vi "PPWV Partial Pressure of Water Vapor (Pa) Pressure Dependent.vi"(1 "Pressure":dbl[unit], 2 "Tceg":dbl[unit], 3 "RH":dbl) -> (0 "PPWV":dbl[unit])   [LabVIEW 2018]
panel:
  out "RH":dbl(knob) scale=0.0..10.0
  out "Pressure":dbl[unit](knob)
  out "PPWV\nPartial Presure of Water Vapor (Pa) Pressure Dependent;\nPPWV=(SVP*RH)/100;":dbl[unit](knob)
  out "Temprature Of Input Air\nKelvin Degree":dbl[unit](slide) scale=273.0..373.0
  out "Tk":dbl[unit]
  out "Temprature Of Input Air\nCentigrade Degree":dbl[unit](slide) scale=0.0..100.0
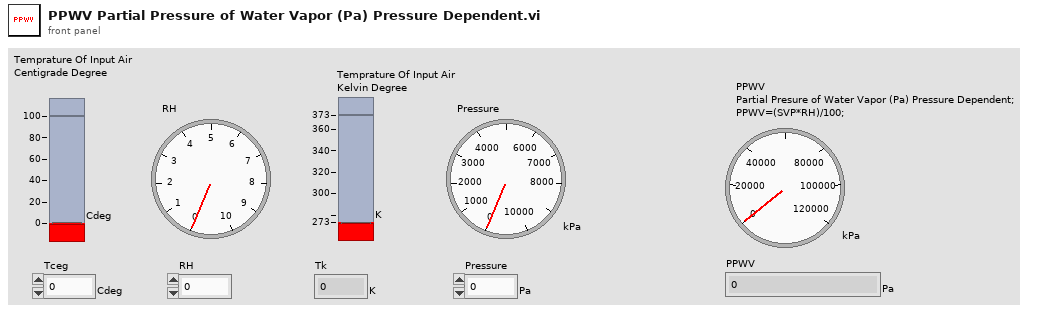
[diagram p1: front panel]
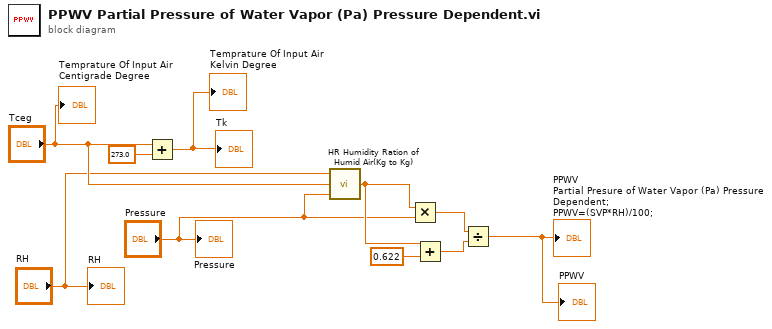
[diagram p0: block diagram]
diagram:
  n1 = Add(x="Tceg", y=dbl[unit] 273.0) -> (x+y=→"Tk" →"Temprature Of Input Air\nKelvin Degree":dbl[unit])
  n2 = call "HR Humidity Ration of Humid Air(Kg to Kg).vi"("Gas Presure"="Pressure", "Tceg"="Tceg", "RH"="RH") -> ("HR"=w3:dbl)
  n3 = Multiply(x=w3, y="Pressure") -> (x*y=w8:dbl[unit])
  n4 = Add(x=w3, y=0.622) -> (x+y=w7:dbl)
  n5 = Divide(x=w8, y=w7) -> (x/y=→"PPWV\nPartial Presure of Water Vapor (Pa) Pressure Dependent;\nPPWV=(SVP*RH)/100;" →"PPWV":dbl[unit])
  "Temprature Of Input Air\nCentigrade Degree" <- "Tceg"
  "Pressure" <- "Pressure"
  "RH" <- "RH"
